vi "Create directory from file path.vi"(8 "error in (no error)":errorcluster, 10 "File path":string, 11 "File Transfer Behavior in":refnum<class "File Transfer Behavior.lvclass">) -> (0 "error out":errorcluster, 3 "File Transfer Behavior out":refnum<class "File Transfer Behavior.lvclass">)   [LabVIEW 2015, in "RT Management.lvlib" / "File Transfer Behavior.lvclass"]
doc: "Creates the directory or directories needed to place a file there.\n\nFor example, if \"File path\" is \"/dir1/dir2/file\", this VI ensures that the directory \"/dir1/dir2\" is created."
uses:
  File Transfer Behavior.lvclass
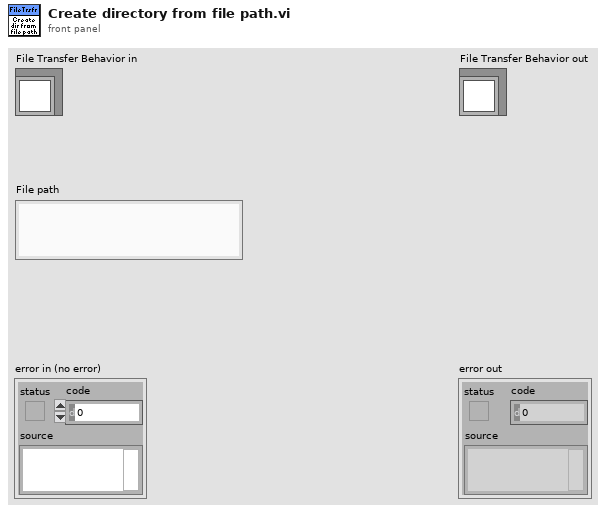
[diagram p1: front panel]
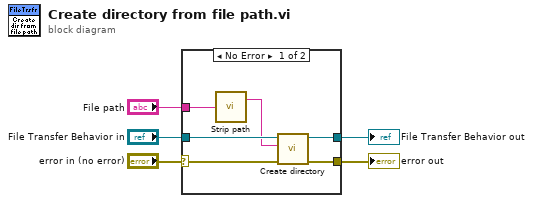
[diagram p0: block diagram]
diagram:
  n1 = case shown="No Error" "error in (no error)" {
    selector: "error in (no error)" -> [w11 w13]
    tunnel: [w10 w13] -> w4
    tunnel: [w9 w12] -> w2
    tunnel: "File Transfer Behavior in" -> [w8 w12]
    tunnel: "File path" -> [w7 _]
    frame No Error {
      n2 = call "Strip path.vi"("Path"=w7) -> ("Stripped path"=w6:string)  [unwired: 2 in, 1 out]
      n3 = call-dynamic "Create directory.vi"("error in (no error)"=w11, "Directory"=w6, "File Transfer Behavior in"=w8) -> ("error out"=w10:errorcluster, "File Transfer Behavior out"=w9:refnum<class "File Transfer Behavior.lvclass">)  [unwired: 7 in]
    }
    frame Error {
    }
  }
  "error out" <- w4
  "File Transfer Behavior out" <- w2
